vi "周期设置_CODMn.vi"() -> ()   [LabVIEW 2016, in "斯坦道CODMn.lvlib"]
uses:
  <vilib>/Utility/miscctls.llb/LVPointTypeDef.ctl
  <vilib>/Utility/config.llb/NI_LVConfig.lvlib
panel:
  in  "运行周期":T1={"运行模式"=enum."维护模式", "质控频次"=enum."关闭", "空白核查时间"=2, "跨度核查时间"=6, "24H周期设置"=4} {"跨度核查时间" items=["00H", "01H", "02H", "03H", "04H", "05H", "06H", "07H", "08H", "09H", "10H", "11H", "12H", "13H", "14H", "15H", "16H", "17H", "18H", "19H", "20H", "21H", "22H", "23H", "关闭"]; "空白核查时间" items=["00H", "01H", "02H", "03H", "04H", "05H", "06H", "07H", "08H", "09H", "10H", "11H", "12H", "13H", "14H", "15H", "16H", "17H", "18H", "19H", "20H", "21H", "22H", "23H", "关闭"]}
  # "运行模式："
  # "质控频次："
  # "空白核查时间："
  # "跨度核查时间："
  # "启动间隔："
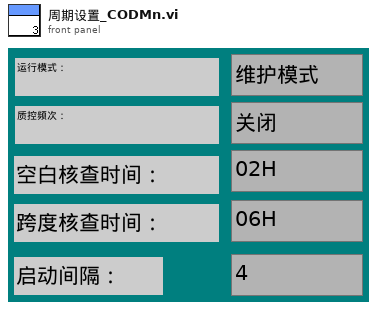
[diagram p1: front panel]
types:
  T1 = cluster{"运行模式":enum16{"维护模式", "常规模式", "应急模式", "质控模式"}, "质控频次":enum16{"关闭", "每天", "星期一", "星期二", "星期三", "星期四", "星期五", "星期六", "星期日"}, "空白核查时间":u16, "跨度核查时间":u16, "24H周期设置":u16}
  T2 = typedef "LVPointTypeDef.ctl" = cluster{"Horizontal":i16, "Vertical":i16}
  T3 = cluster{"测量模式":enum16{"水样测量", "标样核查", "零点核查", "跨度核查", "空白测试", "加标回收", "平行样", "校零", "校标"}}
  T4 = enum16{"关闭", "每天", "星期一", "星期二", "星期三", "星期四", "星期五", "星期六", "星期日"}
  T5 = typedef "LVDateTimeRec.ctl" = cluster{"秒数的小数部分":dbl, "秒":i32, "分":i32, "时":i32, "日":i32, "月":i32, "年":i32, "天数（周）":i32, "天数（年）":i32, "DST":i32}
  T6 = cluster{"运行模式":enum16{"维护模式", "常规模式", "应急模式", "质控模式"}, "质控频次":enum16{"关闭", "每天", "星期一", "星期二", "星期三", "星期四", "星期五", "星期六", "星期日"}, "空白核查时间":u16, "跨度核查时间":u16, "测量间隔":u16}
  T7 = typedef "NI_LVConfig.lvlib/Config Data RefNum.ctl" = refnum<k1>
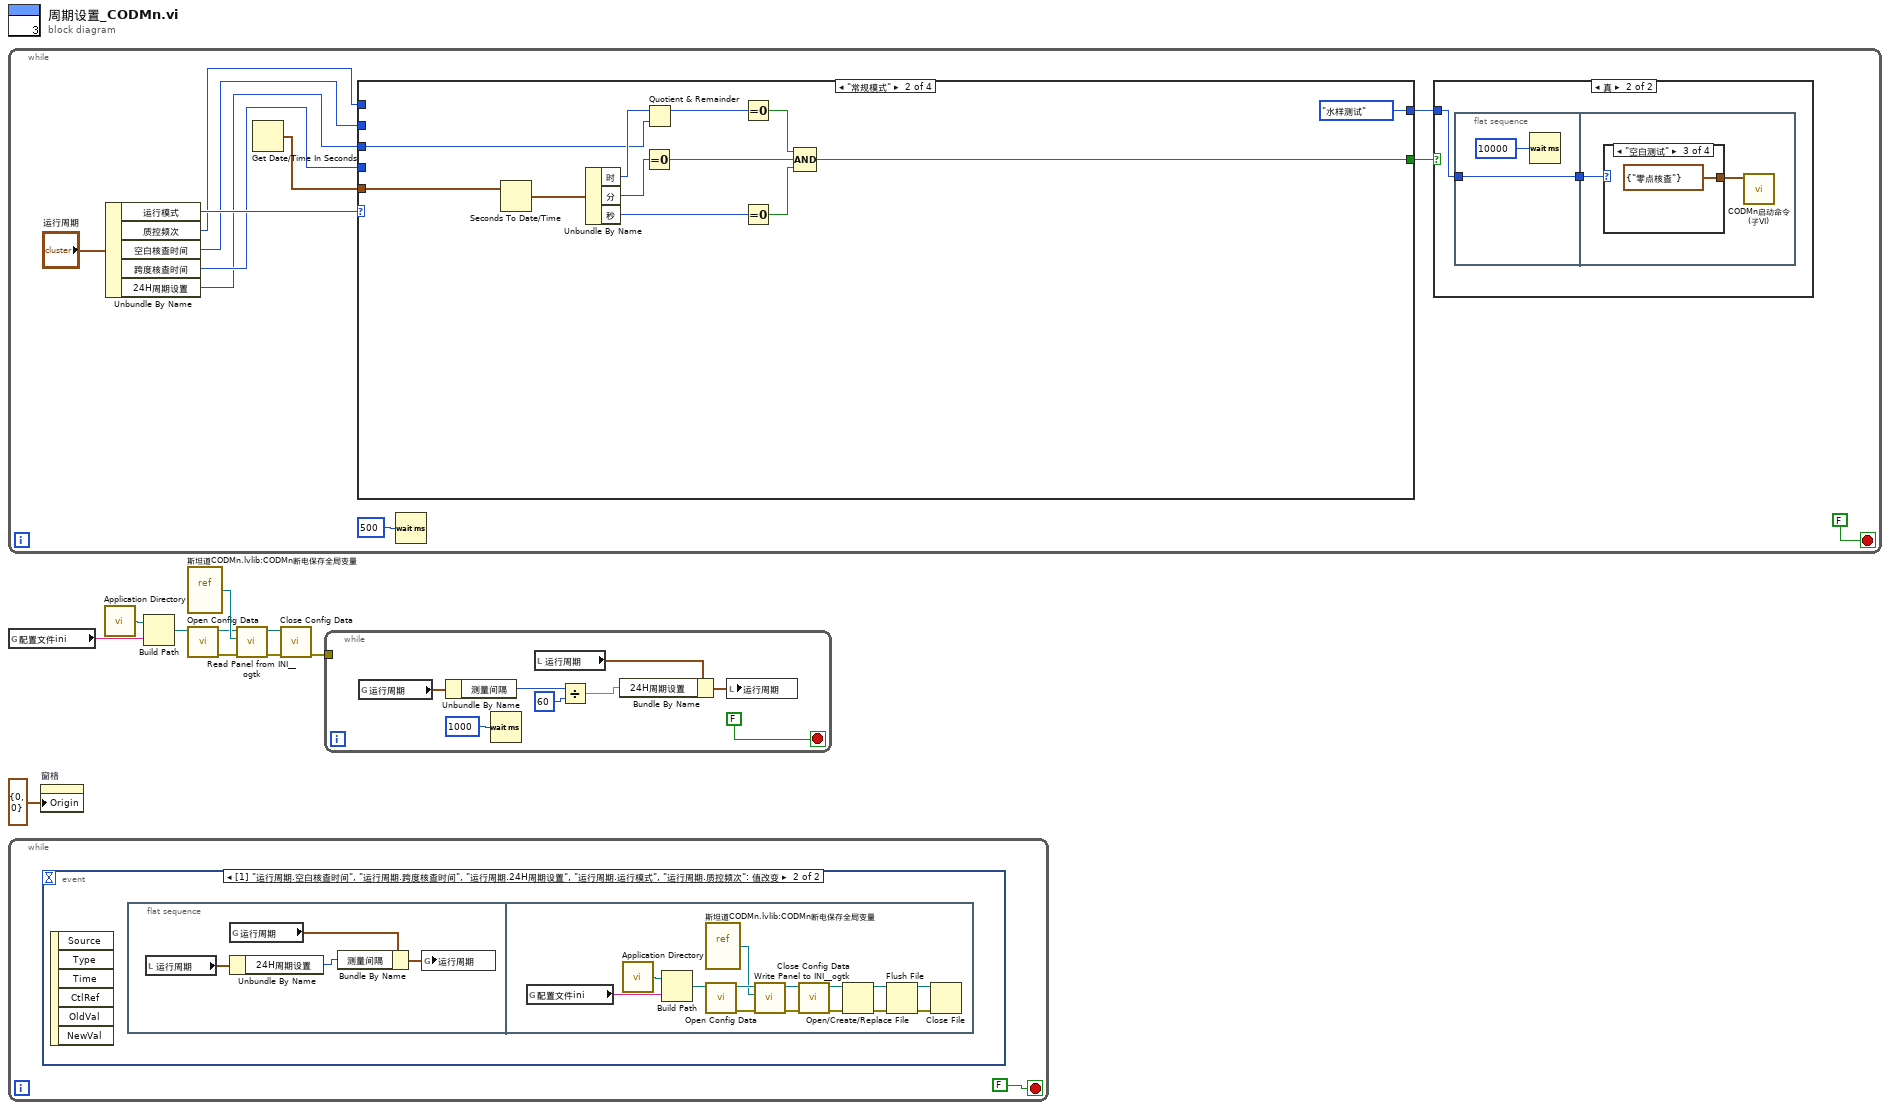
[diagram p0: block diagram]
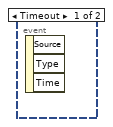
[diagram p2: hidden frame]
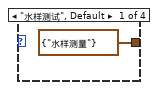
[diagram p4: hidden frame]
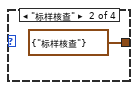
[diagram p5: hidden frame]
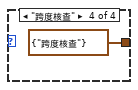
[diagram p6: hidden frame]
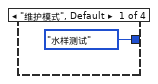
[diagram p7: hidden frame]
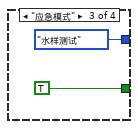
[diagram p8: hidden frame]
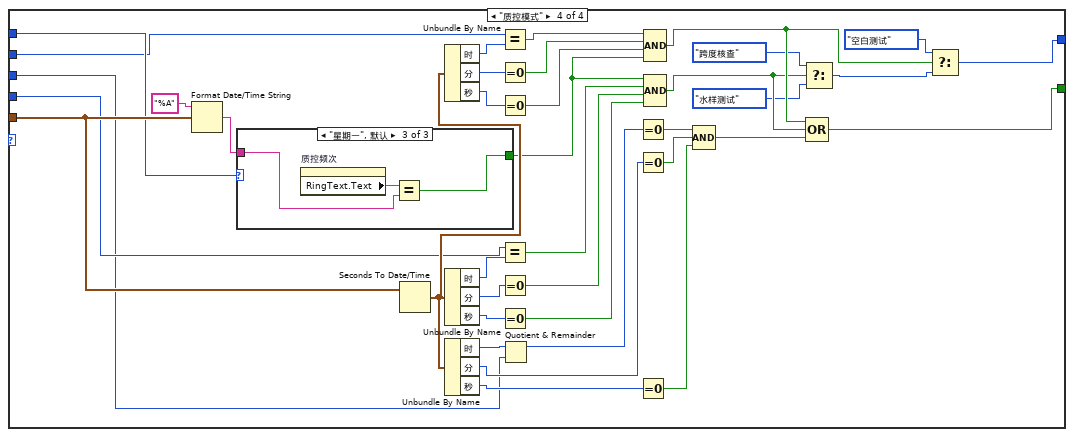
[diagram p9: hidden frame]
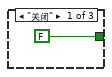
[diagram p10: hidden frame]
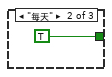
[diagram p11: hidden frame]
diagram:
  n1 = while {
    stop <- FALSE stop-if-true
    n2 = Unbundle By Name("运行周期") -> ("运行模式"=w17:enum16{"维护模式", "常规模式", "应急模式", "质控模式"}, "质控频次"=w16:T4, "空白核查时间"=w15:u16, "跨度核查时间"=w14:u16, "24H周期设置"=w13:u16)
    n3 = Get Date/Time In Seconds() -> (seconds since 1Jan1904=w21:timestamp)
    n4 = case shown="\"常规模式\"" w17 {
      tunnel: w21 -> [_ w43 _ w83]
      tunnel: w13 -> [_ w34 _ w47]
      tunnel: [_ w37 TRUE w63] -> w12
      tunnel: [enum16{"水样测试", "标样核查", "空白测试", "跨度核查"}."水样测试" ("仪器测试类型") enum16{"水样测试", "标样核查", "空白测试", "跨度核查"}."水样测试" ("仪器测试类型") enum16{"水样测试", "标样核查", "空白测试", "跨度核查"}."水样测试" ("仪器测试类型") w56] -> w11
      tunnel: w16 -> [_ _ _ w53]
      tunnel: w15 -> [_ _ _ w52]
      tunnel: w14 -> [_ _ _ w51]
      frame "维护模式", Default {
      }
      frame "常规模式" {
        n5 = Seconds To Date/Time(time stamp (now)=w43) -> (date time rec=w42:T5)  [unwired: 1 in]
        n6 = Unbundle By Name(w42) -> ("时"=w35:i32, "分"=w41:i32, "秒"=w40:i32)
        n7 = Equal To 0?(x=w41) -> (x = 0?=w39:bool)
        n8 = Quotient & Remainder(x=w35, y=w34) -> (x-y*floor(x/y)=w36:i32)  [unwired: 1 out]
        n9 = Equal To 0?(x=w36) -> (x = 0?=w33:bool)
        n10 = Equal To 0?(x=w40) -> (x = 0?=w38:bool)
        n11 = Compound Arithmetic op=AND ("复合运算")(w33, w39, w38) -> (w37:bool)
      }
      frame "应急模式" {
      }
      frame "质控模式" {
        n12 = Format Date/Time String(time format string (%c)="%A" ("时间格式字符串(%c)"), seconds (now)=w83) -> (date/time string=w81:string)  [unwired: 1 in]
        n13 = case shown="\"星期一\", 默认" w53 {
          tunnel: w81 -> [_ _ w87]
          tunnel: [FALSE TRUE w86] -> w54
          frame "关闭" {
          }
          frame "每天" {
          }
          frame "星期一", Default {
            n14 = property on="质控频次" class="Enum (严格)"() -> ("RingText.Text"=w88:string)  [unwired: 2 in, 2 out]
            n15 = Equal?(x=w88, y=w87) -> (x = y?=w86:bool)
          }
        }
        n16 = Seconds To Date/Time(time stamp (now)=w83) -> (date time rec=w67:T5)  [unwired: 1 in]
        n17 = Unbundle By Name(w67) -> ("时"=w76:i32, "分"=w75:i32, "秒"=w74:i32)
        n18 = Unbundle By Name(w67) -> ("时"=w68:i32, "分"=w69:i32, "秒"=w70:i32)
        n19 = Unbundle By Name(w67) -> ("时"=w48:i32, "分"=w80:i32, "秒"=w78:i32)
        n20 = Equal?(x=w52, y=w76) -> (x = y?=w73:bool)
        n21 = Equal To 0?(x=w75) -> (x = 0?=w72:bool)
        n22 = Equal To 0?(x=w74) -> (x = 0?=w71:bool)
        n23 = Equal?(x=w51, y=w68) -> (x = y?=w66:bool)
        n24 = Equal To 0?(x=w69) -> (x = 0?=w65:bool)
        n25 = Equal To 0?(x=w70) -> (x = 0?=w64:bool)
        n26 = Quotient & Remainder(x=w48, y=w47) -> (x-y*floor(x/y)=w50:i32)  [unwired: 1 out]
        n27 = Equal To 0?(x=w50) -> (x = 0?=w49:bool)
        n28 = Equal To 0?(x=w80) -> (x = 0?=w79:bool)
        n29 = Equal To 0?(x=w78) -> (x = 0?=w77:bool)
        n30 = Compound Arithmetic op=AND ("复合运算")(w73, w72, w71, w54) -> (w62:bool)
        n31 = Compound Arithmetic op=AND ("复合运算")(w54, w66, w65, w64) -> (w60:bool)
        n32 = Compound Arithmetic op=AND ("复合运算")(w49, w79, w77) -> (w55:bool)
        n33 = Select(t=enum16{"水样测试", "标样核查", "空白测试", "跨度核查"}."跨度核查" ("仪器测试类型"), s=w60, f=enum16{"水样测试", "标样核查", "空白测试", "跨度核查"}."水样测试" ("仪器测试类型")) -> (s? t:f=w58:enum16{"水样测试", "标样核查", "空白测试", "跨度核查"})
        n34 = Compound Arithmetic op=OR ("复合运算")(w62, w60, w55) -> (w63:bool)
        n35 = Select(t=enum16{"水样测试", "标样核查", "空白测试", "跨度核查"}."空白测试" ("仪器测试类型"), s=w62, f=w58) -> (s? t:f=w56:enum16{"水样测试", "标样核查", "空白测试", "跨度核查"})
      }
    }
    n36 = Wait (ms)(milliseconds to wait=u32 500 ("等待时间（毫秒）")) -> ()  [unwired: 1 out]
    n37 = case shown="真" w12 {
      tunnel: w11 -> [_ w23]
      frame False {
      }
      frame True {
        n38 = flat-sequence {
          tunnel: w23 -> [w25]
          tunnel: [w25] -> w22
          tunnel: w22 -> [w27]
          frame #0 {
            n39 = Wait (ms)(milliseconds to wait=u32 10000 ("等待时间（毫秒）")) -> ()  [unwired: 1 out]
          }
          frame #1 {
            n40 = case shown="\"空白测试\"" w27 {
              tunnel: [T3 {"测量模式"=enum."水样测量"} ("启动测量模式") T3 {"测量模式"=enum."标样核查"} ("启动测量模式") T3 {"测量模式"=enum."零点核查"} ("启动测量模式") T3 {"测量模式"=enum."跨度核查"} ("启动测量模式")] -> w26
              frame "水样测试", Default {
              }
              frame "标样核查" {
              }
              frame "空白测试" {
              }
              frame "跨度核查" {
              }
            }
            n41 = call "CODMn启动命令 (子VI).vi"("启动测量模式"=w26) -> ()  [unwired: 11 in]
          }
        }
      }
    }
  }
  n42 = global read "COD内部交互全局.vi" "配置文件ini"() -> (w1:string)
  n43 = while {
    stop <- FALSE stop-if-true
    n44 = event shown="[1] \"运行周期.空白核查时间\", \"运行周期.跨度核查时间\", \"运行周期.24H周期设置\", \"运行周期.运行模式\", \"运行周期.质控频次\": 值改变" {
      selector: _ -> [_ _]
      dyn-events: _ -> [_ _]
      timeout: _ -> [_ _]
      event Timeout {
        n45 = event-data() -> ()  [unwired: 1 in, 3 out]
      }
      event "运行周期.空白核查时间", "运行周期.跨度核查时间", "运行周期.24H周期设置", "运行周期.运行模式", "运行周期.质控频次": Value Change {
        n46 = event-data() -> ()  [unwired: 1 in, 6 out]
        n47 = flat-sequence {
          frame #0 {
            n48 = local read "运行周期"() -> (w93:T1)
            n49 = global read "CODMn断电保存全局变量.vi" "运行周期"() -> (w92:T6)
            n50 = Unbundle By Name(w93) -> ("24H周期设置"=w90:u16)
            n51 = Bundle By Name(cluster=w92, "测量间隔"=w90) -> (w91:T6)
            n52 = global write "CODMn断电保存全局变量.vi" "运行周期"(w91) -> ()
          }
          frame #1 {
            n53 = global read "COD内部交互全局.vi" "配置文件ini"() -> (w94:string)
            n54 = call <vilib>:"Application Directory.vi"() -> ("Application Directory"=w107:path)
            n55 = Build Path(base path=w107, name or relative path=w94) -> (appended path=w106:path)
            n56 = vi-ref "斯坦道CODMn.lvlib:CODMn断电保存全局变量.vi"() -> (w104:refnum<vi>)
            n57 = call <vilib>:"Open Config Data.vi"("configuration file path"=w106) -> ("error out"=w102:errorcluster, "refnum"=w105:T7)  [unwired: 8 in, 1 out]
            n58 = call <userlib>:"Write Panel to INI__ogtk.vi"("error in (no error)"=w102, "VI ref"=w104, "refnum"=w105) -> ("error out"=w101:errorcluster, "refnum out"=w103:T7)  [unwired: 7 in]
            n59 = call <vilib>:"Close Config Data.vi"("error in (no error)"=w101, "refnum"=w103) -> ("error out"=w96:errorcluster, "file path"=w95:path)  [unwired: 8 in]
            n60 = Open/Create/Replace File(file path (use dialog)=w95, error in=w96) -> (refnum out=w99:refnum<file>, error out=w100:errorcluster)  [unwired: 4 in, 1 out]
            n61 = Flush File(refnum=w99, error in=w100) -> (refnum out=w98:refnum<file>, error out=w97:errorcluster)
            n62 = Close File(refnum=w98, error in=w97) -> ()  [unwired: 2 out]
          }
        }
      }
    }
  }
  n63 = property on="窗格" class="Pane"("Origin"=T2 {"Horizontal"=0, "Vertical"=0} ("原点")) -> ()  [unwired: 2 in, 2 out]
  n64 = call <vilib>:"Application Directory.vi"() -> ("Application Directory"=w4:path)
  n65 = Build Path(base path=w4, name or relative path=w1) -> (appended path=w5:path)
  n66 = vi-ref "斯坦道CODMn.lvlib:CODMn断电保存全局变量.vi"() -> (w7:refnum<vi>)
  n67 = call <vilib>:"Open Config Data.vi"("configuration file path"=w5) -> ("error out"=w9:errorcluster, "refnum"=w6:T7)  [unwired: 8 in, 1 out]
  n68 = call <userlib>:"Read Panel from INI__ogtk.vi"("error in (no error)"=w9, "VI ref"=w7, "refnum"=w6) -> ("error out"=w10:errorcluster, "refnum out"=w8:T7)  [unwired: 7 in]
  n69 = call <vilib>:"Close Config Data.vi"("error in (no error)"=w10, "refnum"=w8) -> ("error out"=w3:errorcluster)  [unwired: 8 in, 1 out]
  n70 = while {
    tunnel: w3 -> [_]
    stop <- FALSE stop-if-true
    n71 = global read "CODMn断电保存全局变量.vi" "运行周期"() -> (w113:T6)
    n72 = Unbundle By Name(w113) -> ("测量间隔"=w112:u16)
    n73 = Wait (ms)(milliseconds to wait=u32 1000 ("等待时间（毫秒）")) -> ()  [unwired: 1 out]
    n74 = local read "运行周期"() -> (w109:T1)
    n75 = Divide(x=w112, y=u16 60) -> (x/y=w108:dbl)
    n76 = Bundle By Name(cluster=w109, "24H周期设置"=w108) -> (w110:T1)
    n77 = local write "运行周期"(w110) -> ()
  }
